vi "FTW-Ether-Logger-Construct.vi"(5 "FTW Ether Configuration":string="{\n  \"ApplicationName\": \"Featherweight Application\",\n  \"ApplicationVersion\": \"0.1.0-1\",\n  \"LoggerAddress\": \"inproc://*\",\n  \"LoggerName\": \"Log\",\n  \"LoggerDirectory\": \"[UserAppData]\\\\Featherweight\\\\Logs\",\n  \"LoggerDiskThrashDelay\": 200\n}", 11 "error in":errorcluster) -> (15 "error out":errorcluster)   [LabVIEW 2015, in "FTW-Ether.lvclass"]
uses:
  FTW-Ether.lvclass
  JSON/FTW-JSON-JoinMode.ctl
  FTW-Ether-Instance.vi
  EventLogger/FTW-Logger.lvclass
  container/FTW-Container.lvclass
panel:
  # "Inputs"
  # "Outputs"
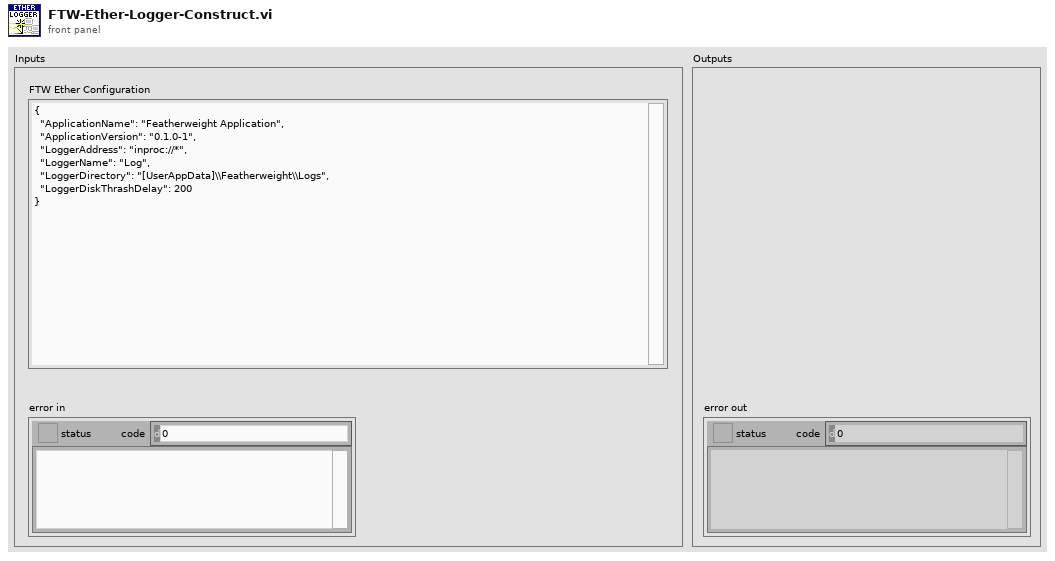
[diagram p1: front panel]
types:
  T1 = typedef "FTW-JSON-JoinMode.ctl" = enum32{"Upsert", "Update Only", "Insert Only"}
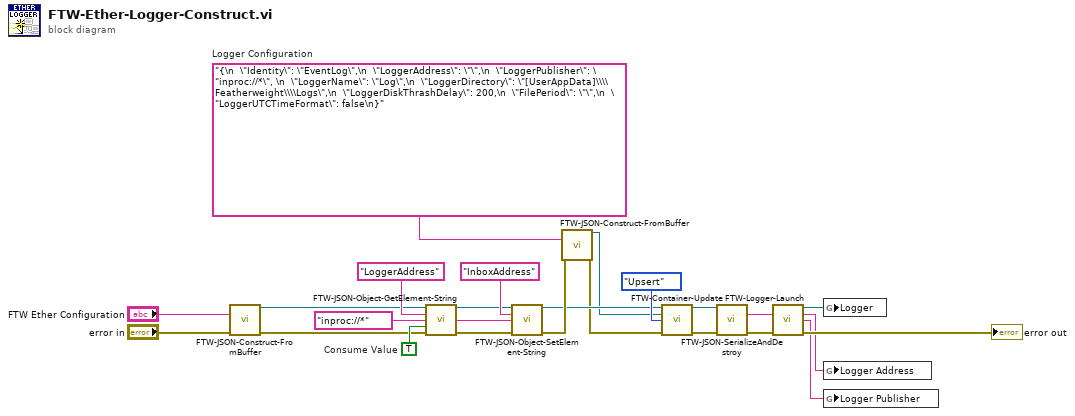
[diagram p0: block diagram]
diagram:
  w4 = "{\n  \"Identity\": \"EventLog\",\n  \"LoggerAddress\": \"\",\n  \"LoggerPublisher\": \"inproc://*\", \n  \"LoggerName\": \"Log\",\n  \"LoggerDirectory\": \"[UserAppData]\\\\Featherweight\\\\Logs\",\n  \"LoggerDiskThrashDelay\": 200,\n  \"FilePeriod\": \"\",\n  \"LoggerUTCTimeFormat\": false\n}"  # Logger Configuration
  w14 = TRUE  # Consume Value
  n1 = call "FTW-JSON-Construct-FromBuffer.vi"("JSON String (UTF-8)"="FTW Ether Configuration", "error in"="error in") -> ("JSON"=w9:refnum<class "FTW-Container.lvclass">, "error out"=w10:errorcluster)  [unwired: 12 in]
  n2 = call "FTW-JSON-Object-GetElement-String.vi"("JSON"=w9, "Key"="LoggerAddress", "Default Value"="inproc://*", "Consume Value"=w14, "error in"=w10) -> ("JSON out"=w8:refnum<class "FTW-Container.lvclass">, "Value"=w12:string, "error out"=w17:errorcluster)  [unwired: 6 in, 2 out]
  n3 = call "FTW-JSON-Object-SetElement-String.vi"("JSON"=w8, "Key"="InboxAddress", "Value"=w12, "error in"=w17) -> ("JSON out"=w7:refnum<class "FTW-Container.lvclass">, "error out"=w13:errorcluster)  [unwired: 10 in]
  n4 = call "FTW-JSON-Construct-FromBuffer.vi"("JSON String (UTF-8)"=w4, "error in"=w13) -> ("JSON"=w5:refnum<class "FTW-Container.lvclass">, "error out"=w6:errorcluster)  [unwired: 12 in]
  n5 = call "FTW-Container-Update.vi"("FTW-Container In"=w7, "Other Container"=w5, "Join Mode"=FTW-JSON-JoinMode."Upsert" ("Update Mode (0: Upsert)"), "error in"=w6) -> ("Updated Container"=w2:refnum<class "FTW-Container.lvclass">, "error out"=w19:errorcluster)  [unwired: 10 in]
  n6 = call "FTW-JSON-SerializeAndDestroy.vi"("JSON"=w2, "error in"=w19) -> ("JSON String (UTF-8)"=w1:string, "error out"=w3:errorcluster)  [unwired: 12 in]
  n7 = call "FTW-Logger-Launch.vi"("FTW Logger Configuration"=w1, "error in"=w3) -> ("FTW Logger Connector"=w22:refnum<class "FTW-Logger.lvclass">, "Logger Address"=w21:string, "Publisher Address"=w20:string, "error out"=→"error out":errorcluster)  [unwired: 10 in]
  n8 = global write "FTW-Ether-Instance.vi" "Logger"(w22) -> ()
  n9 = global write "FTW-Ether-Instance.vi" "Logger Address"(w21) -> ()
  n10 = global write "FTW-Ether-Instance.vi" "Logger Publisher"(w20) -> ()
